vi "Configure Measurement (ACP).vi"(0 "VISA resource name":refnum<visa-resource-name>, 1 "Enable Noise Correction (F: Disable)":bool, 2 "Enable Limit Test (F: Disable)":bool, 5 "Measurement Type (0: Total Power Reference)":i32(ring) items=["Total Power Reference", "PSD Reference"], 9 "Measurement Method (0: Integration BW)":i32(ring) items=["Integration Bandwidth", "Filtered IBW (max dynamic range)", "RBW", "Fast"], 11 "error in (no error)":errorcluster, 12 "Bandwidth Filter Type (0: Gaussian)":i32(ring) items=["Gaussian", "Flattop"]) -> (4 "VISA resource name out":refnum<visa-resource-name>, 15 "error out":errorcluster)   [LabVIEW 2014, in "Agilent MXA Series.lvlib"]
doc: "Sets the ACP measurement parameters."
uses:
  Agilent MXA Series.lvlib
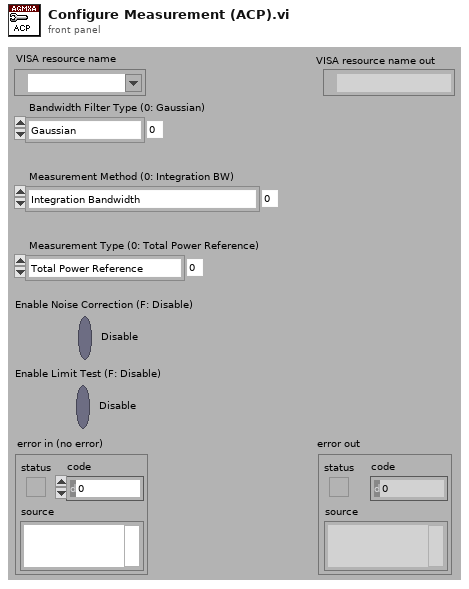
[diagram p1: front panel]
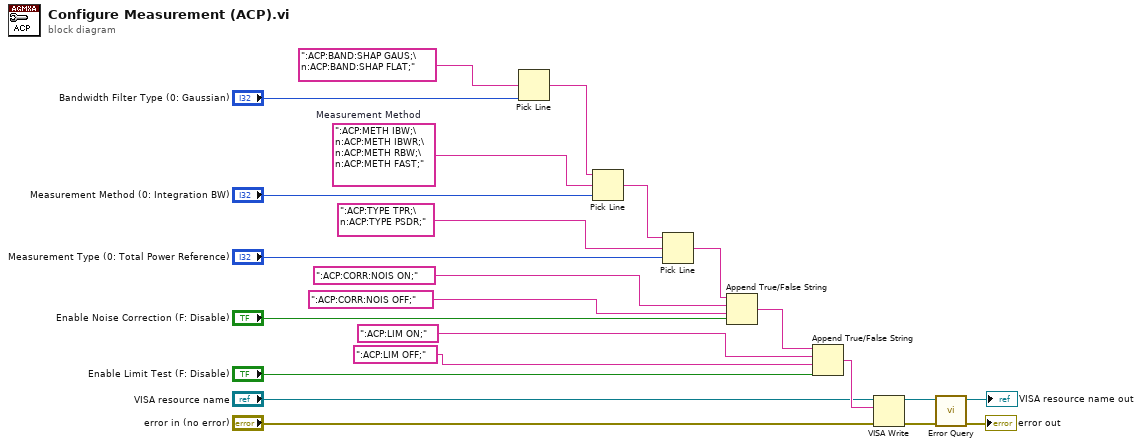
[diagram p0: block diagram]
diagram:
  w21 = ":ACP:METH IBW;\n:ACP:METH IBWR;\n:ACP:METH RBW;\n:ACP:METH FAST;"  # Measurement Method
  n1 = Pick Line(multi-line string=":ACP:BAND:SHAP GAUS;\n:ACP:BAND:SHAP FLAT;", line index="Bandwidth Filter Type (0: Gaussian)") -> (output string=w16:string)  [unwired: 1 in]
  n2 = Pick Line(string ("")=w16, multi-line string=w21, line index="Measurement Method (0: Integration BW)") -> (output string=w17:string)
  n3 = Pick Line(string ("")=w17, multi-line string=":ACP:TYPE TPR;\n:ACP:TYPE PSDR;", line index="Measurement Type (0: Total Power Reference)") -> (output string=w10:string)
  n4 = Append True/False String(1:"Enable Noise Correction (F: Disable)", 2:":ACP:CORR:NOIS OFF;" ("false string"), 3:":ACP:CORR:NOIS ON;" ("true string"), 4:w10) -> (0:w9:string)
  n5 = Append True/False String(1:"Enable Limit Test (F: Disable)", 2:":ACP:LIM OFF;" ("false string"), 3:":ACP:LIM ON;" ("true string"), 4:w9) -> (0:w8:string)
  n6 = VISA Write(VISA resource name="VISA resource name", write buffer=w8, error in (no error)="error in (no error)") -> (VISA resource name out=w4:refnum<visa-resource-name>, error out=w5:errorcluster)  [unwired: 1 out]
  n7 = call "Error Query.vi"("error in (no error)"=w5, "VISA resource name"=w4) -> ("error out"=→"error out":errorcluster, "VISA resource name out"=→"VISA resource name out":refnum<visa-resource-name>)  [unwired: 6 in, 2 out]
